vi "DAQmx Self Calibrate.vi"(0 "device in":tag, 11 "error in":errorcluster) -> (15 "error out":errorcluster)   [LabVIEW 2010]
doc: "Measures the onboard reference voltage of the device and adjusts the self-calibration constants to account for any errors caused by short-term fluctuations in the operating environment. When you self-calibrate a device, no external signal connections are necessary."
uses:
  nilvaiu.dll
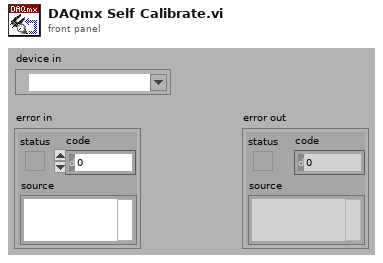
[diagram p1: front panel]
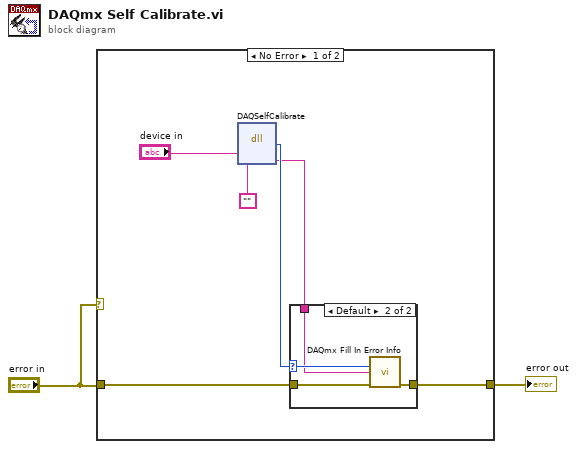
[diagram p0: block diagram]
diagram:
  n1 = case shown="No Error" "error in" {
    tunnel: [w7 w14] -> w1
    tunnel: "error in" -> [w8 w14]
    frame No Error {
      n2 = dll-call lib="nilvaiu.*" fn="DAQSelfCalibrate"("deviceID"="device in", "extendedErrorInfo"="") -> (w6:i32, "extendedErrorInfo"=w5:string)  [unwired: 4 in, 2 out]
      n3 = case shown="Default" w6 {
        selector: w6 -> [_ w11]
        tunnel: w8 -> [w9 w13]
        tunnel: [w9 w12] -> w7
        tunnel: w5 -> [_ w10]
        frame 0 {
        }
        frame Default {
          n4 = call <vilib>:"DAQmx Fill In Error Info.vi"("status code"=w11, "extended error info"=w10, "error in"=w13) -> ("error out"=w12:errorcluster)  [unwired: 12 in]
        }
      }
    }
    frame Error {
    }
  }
  "error out" <- w1
